vi "Tektronix 7000 Series Transfer Current Waveform.vi"() -> ()   [LabVIEW 2015]
doc: "This example illustrates how to transfer the current waveform on an oscilloscope."
uses:
  <instrlib>/Tektronix 7000 Series/Public/Data/Low Level/Fetch (Waveform).vi
  <instrlib>/Tektronix 7000 Series/Tektronix 7000 Series.lvlib
panel:
  in  "Acquisition Type (0:Sample)":u16(ring) items=["Sample", "Peak Detect", "Hi Res", "Average", "Envelope", "WfmDB"]
  in  "Maximum Time (10000ms)":u32=10000
  in  "Channel (0: Channel 1)":u16(ring) format="%#_5f" items=["Channel 1", "Channel 2", "Channel 3", "Channel 4", "Math 1", "Math 2", "Math 3", "Math 4", "Reference 1", "Reference 2", "Reference 3", "Reference 4"]
  in  "VISA Resource Name":refnum<visa-resource-name>
  out "Waveform Graph":waveform(dbl)(graph)
  # "(c) 2006. National Instruments Corporation. ALL RIGHTS RESERVED."
  # "(c) 2006 - 2016 National Instruments Corporation.  ALL RIGHTS RESERVED."
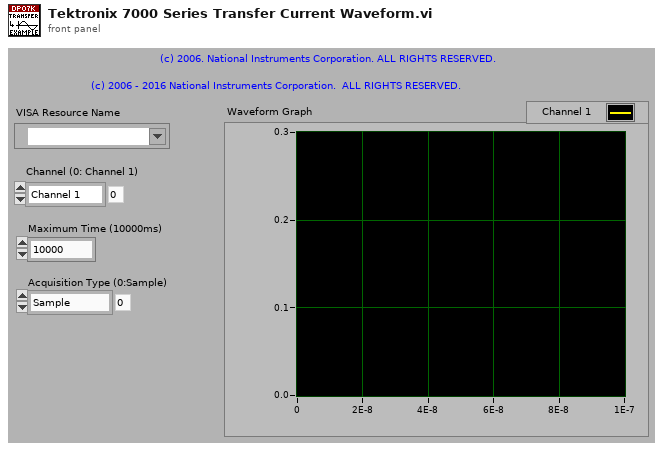
[diagram p1: front panel]
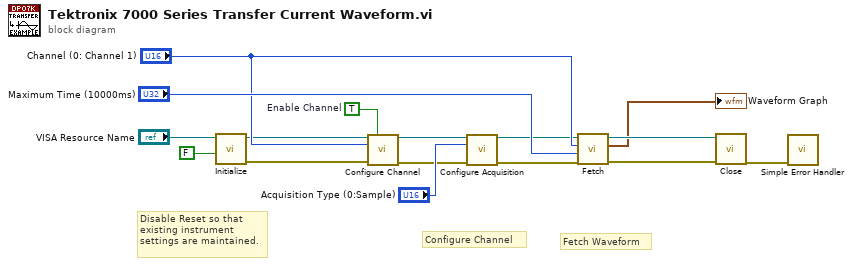
[diagram p0: block diagram]
diagram:
  w1 = TRUE  # Enable Channel
  # "Configure Channel"
  # "Fetch Waveform"
  # "Disable Reset so that \nexisting instrument\nsettings are maintained."
  n1 = call <instrlib>:"Initialize.vi"("Reset? ( Yes)"=FALSE, "VISA resource name"="VISA Resource Name") -> ("error out"=w6:errorcluster, "VISA resource name out"=w7:refnum<visa-resource-name>)  [unwired: 8 in]
  n2 = call <instrlib>:"Configure Channel.vi"("VISA resource name"=w7, "Enable Channel (T: Enable)"=w1, "Channel (0: Channel 1)"="Channel (0: Channel 1)", "error in (no error)"=w6) -> ("VISA resource name out"=w5:refnum<visa-resource-name>, "error out"=w4:errorcluster)  [unwired: 10 in]
  n3 = call <instrlib>:"Configure Acquisition.vi"("VISA resource name"=w5, "Acquisition Type (0:Sample)"="Acquisition Type (0:Sample)", "error in (no error)"=w4) -> ("VISA resource name out"=w3:refnum<visa-resource-name>, "error out"=w2:errorcluster)  [unwired: 11 in]
  n4 = call-poly <instrlib>:"Fetch.vi"("error in (no error)"=w2, "Maximum Time (10000ms)"="Maximum Time (10000ms)", "Channel (0:Channel1)"="Channel (0: Channel 1)", "VISA resource name"=w3) -> ("error out"=w13:errorcluster, "Waveform Data"=→"Waveform Graph":waveform(dbl), "VISA resource name out"=w14:refnum<visa-resource-name>)  [unwired: 5 in]
  n5 = call <instrlib>:"Close.vi"("error in (no error)"=w13, "VISA resource name"=w14) -> ("error out"=w15:errorcluster)  [unwired: 9 in]
  n6 = call <vilib>:"Simple Error Handler.vi"("error in (no error)"=w15) -> ()  [unwired: 4 in, 5 out]
